vi "Dot Edit.vi"() -> ()   [LabVIEW 2019]
uses:
  Classes/Settings/Dot Settings/Dot Settings.lvclass/Dot Settings.ctl
  Classes/Settings/ObjectSettings/ObjectSettings.lvclass/ObjectSettings.ctl
  Classes/Settings/Dot Settings/Dot Settings.lvclass
  C:/Users/Albro/Documents/GitHub/AFM-Lithography/lvsrc/Classes/Settings/ObjectSettings/ObjectSettings.lvclass
  Classes/Settings/Setting Database/Setting Database.lvclass
  Classes/Settings/Setting Database/Typedefs/PrivateEvents--Setting Database.CopyActiveDotToAll.ctl
  <vilib>/JKI/JKI SMO/SMO/SMO.lvclass
  Classes/Settings/Dot Settings/Accessors/Write Action.vi
  Classes/Settings/ObjectSettings/Accessors/Write Enabled.vi
  Classes/Settings/Dot Settings/Accessors/Read Action.vi
  Classes/Settings/ObjectSettings/Accessors/Read Enabled.vi
panel:
  in  "Save Default":bool
  in  "Copy to All":bool
  in  "Action":u16(ring) caption="Ring" items=["Current Voltage", "Quantum Dot"]
  in  "Enabled?":bool=TRUE
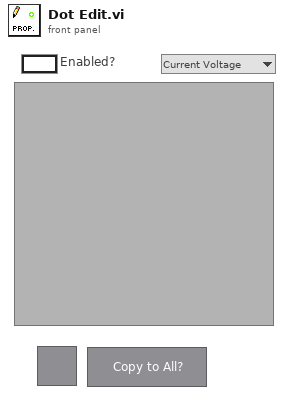
[diagram p1: front panel]
types:
  T1 = enum32{"Invalid", "Standard", "Closed", "Hidden", "Minimized", "Maximized"}
  T2 = enum32{"invalid app kind", "Development System", "Run Time System", "Student Edition", "Embedded LabVIEW", "Evaluation", "Custom"}
  T3 = typedef "Setting Database.lvclass/PrivateEvents--Setting Database.CopyActiveDotToAll.ctl" = bool
  T4 = typedef "Setting Database.lvclass/PublicEvents--Setting Database.NewActiveDot.ctl" = refnum<class "Dot Settings.lvclass">
  T5 = cluster{"Core":cluster{"Current VI Reference":refnum<vi>, "Close Panel on Exit?":bool}, "Active Dot":refnum<class "Dot Settings.lvclass">, "SettingDB":refnum<class "Setting Database.lvclass">, "Subpanels":refnum<vi>[], "Action":u16}
  T6 = cluster{"Current VI Reference":refnum<vi>, "Close Panel on Exit?":bool}
  T7 = typedef "Setting Database.lvclass/PublicEvents--Cluster.ctl" = cluster{"NewActivePath":refnum<user-event>, "PathsUpdated":refnum<user-event>, "RectanglesUpdated":refnum<user-event>, "NewActiveRectangle":refnum<user-event>, "NewActiveFunnel":refnum<user-event>, "FunnelsUpdated":refnum<user-event>, "NewActiveDot":refnum<user-event>, "DotsUpdated":refnum<user-event>}
  T8 = typedef "Dot Settings.lvclass/Action.ctl" = enum16{"IV", "QD"}
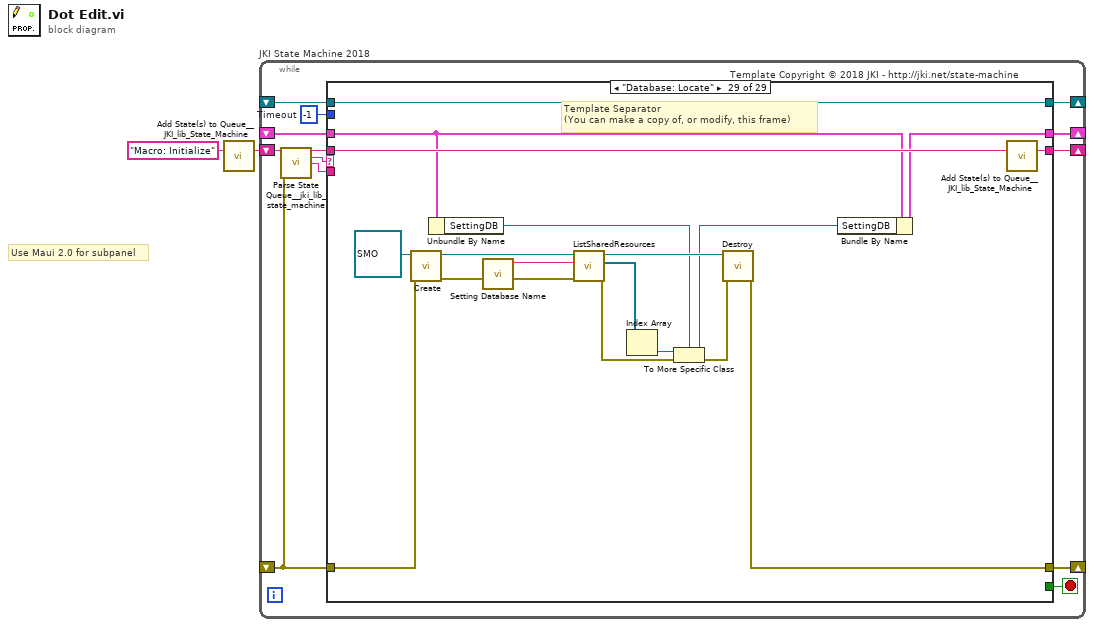
[diagram p0: block diagram]
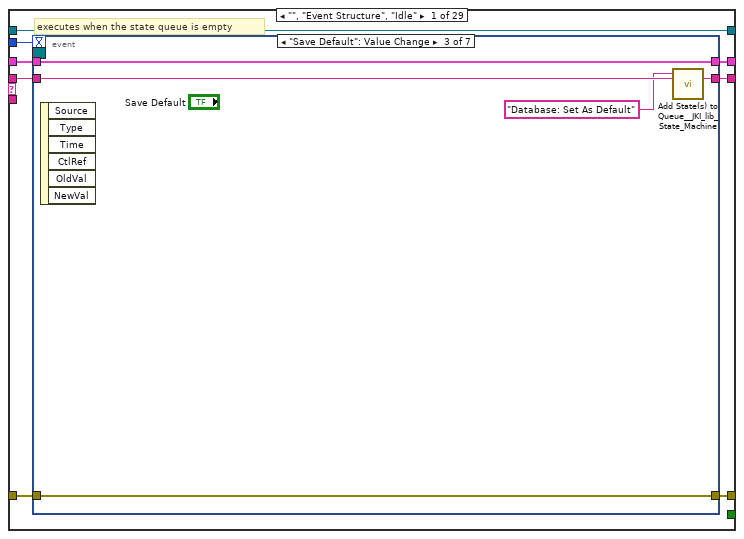
[diagram p2: hidden frame]
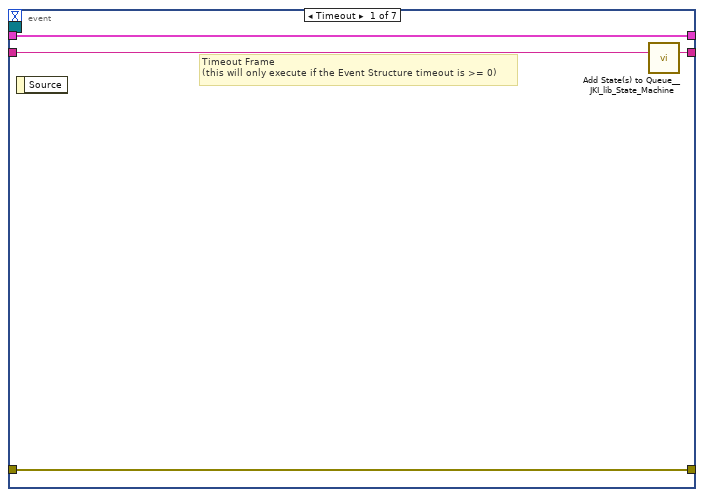
[diagram p3: hidden frame]
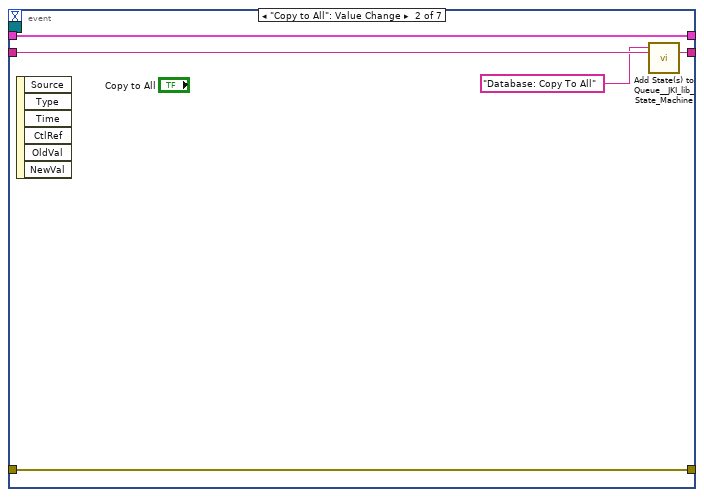
[diagram p4: hidden frame]
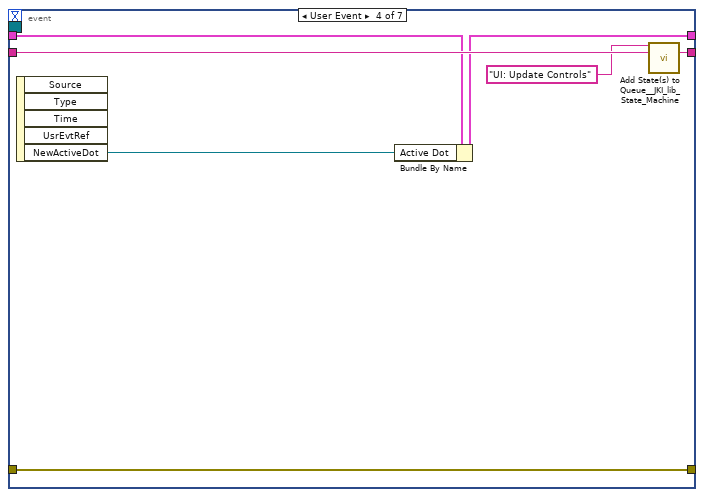
[diagram p5: hidden frame]
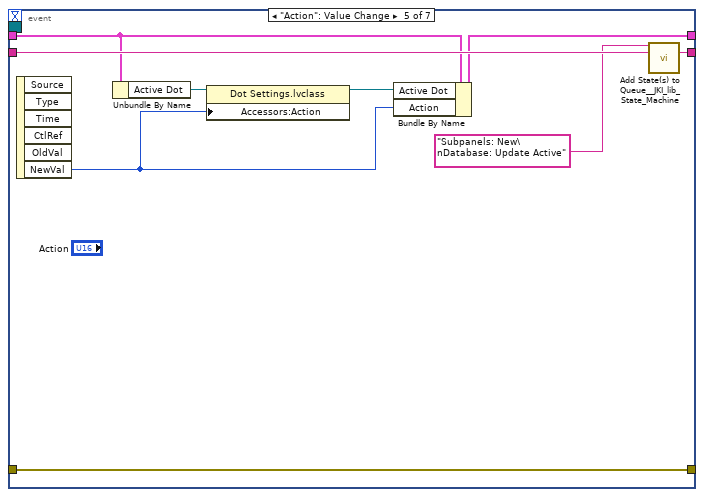
[diagram p6: hidden frame]
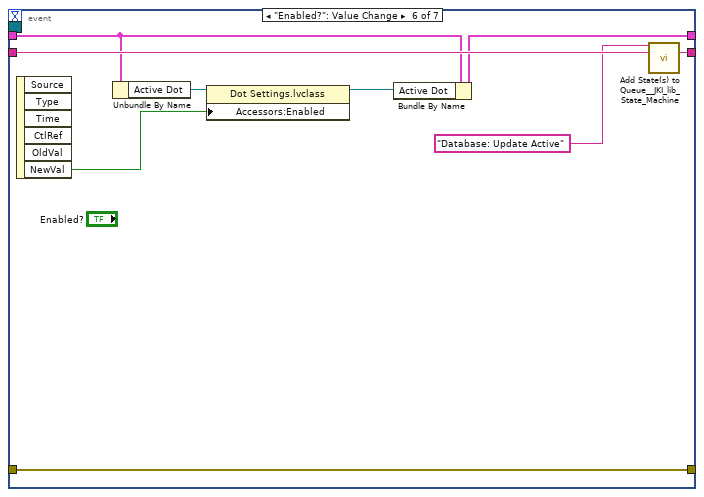
[diagram p7: hidden frame]
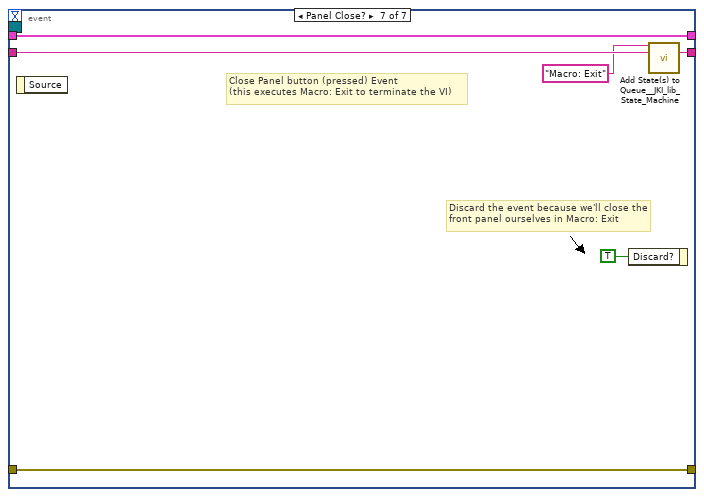
[diagram p8: hidden frame]
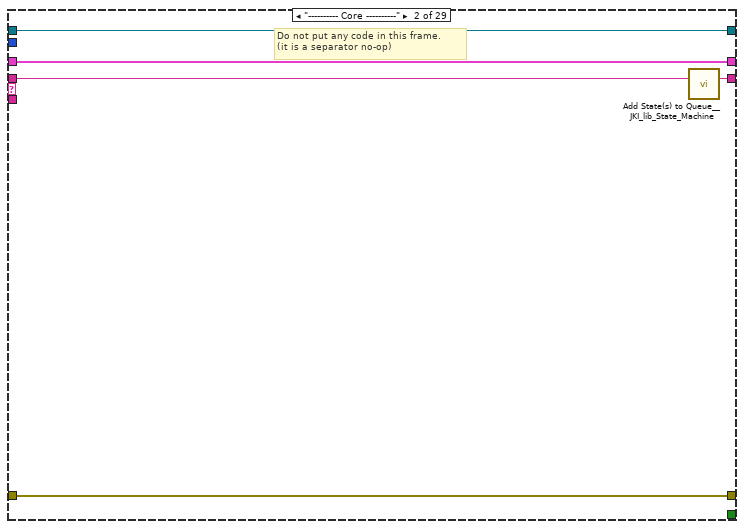
[diagram p9: hidden frame]
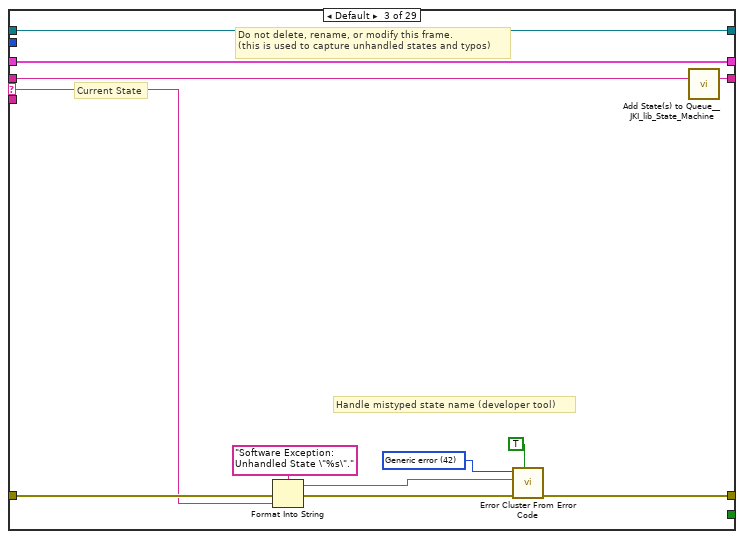
[diagram p10: hidden frame]
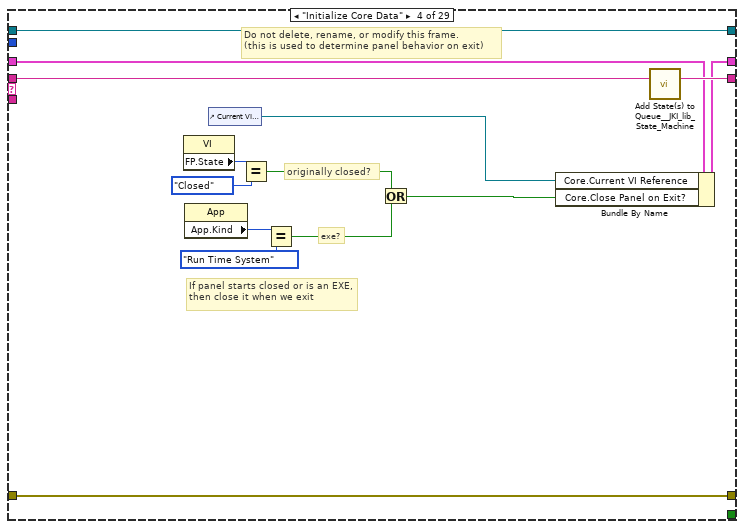
[diagram p11: hidden frame]
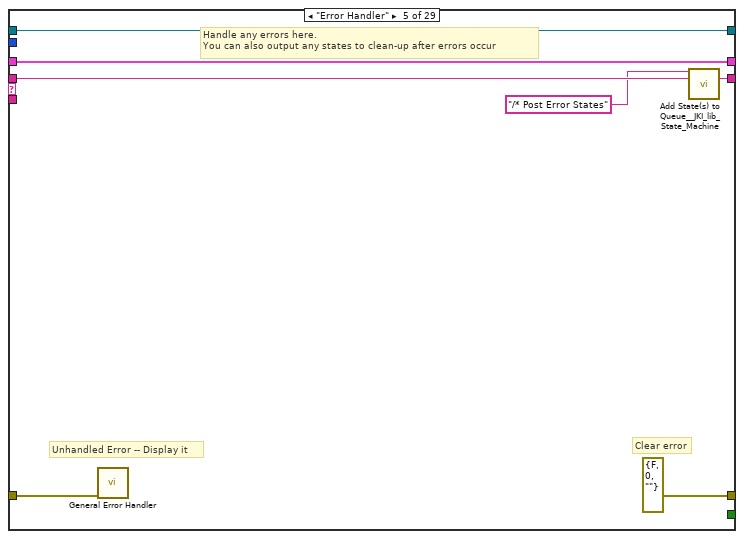
[diagram p12: hidden frame]
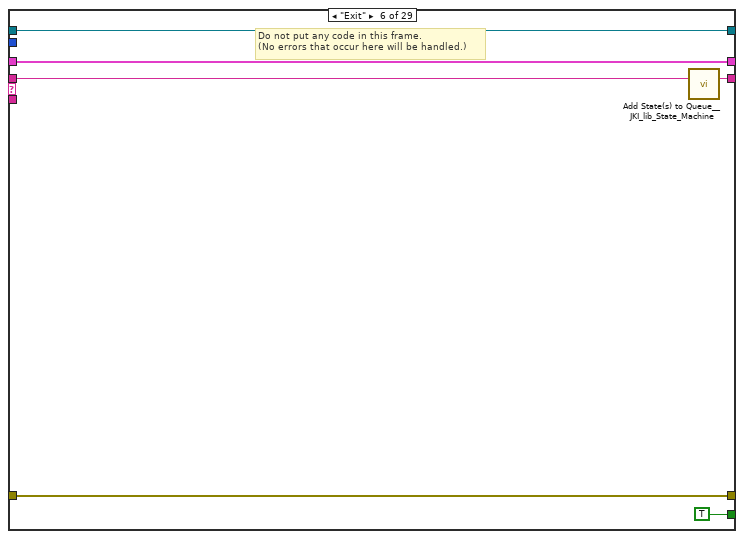
[diagram p13: hidden frame]
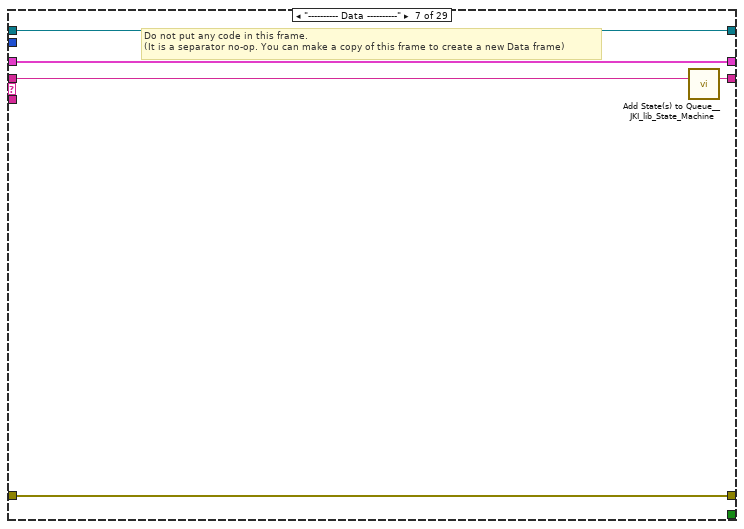
[diagram p14: hidden frame]
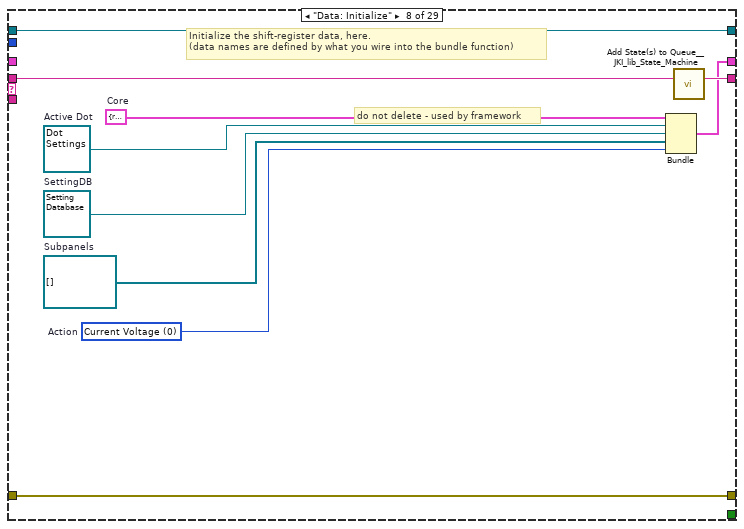
[diagram p15: hidden frame]
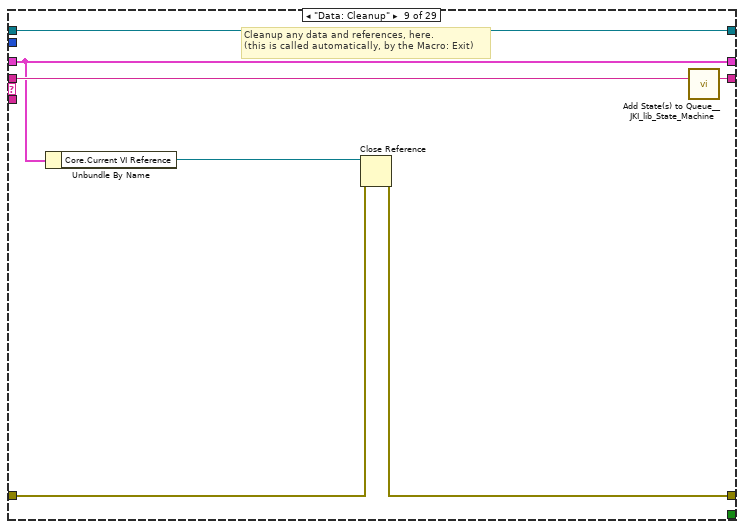
[diagram p16: hidden frame]
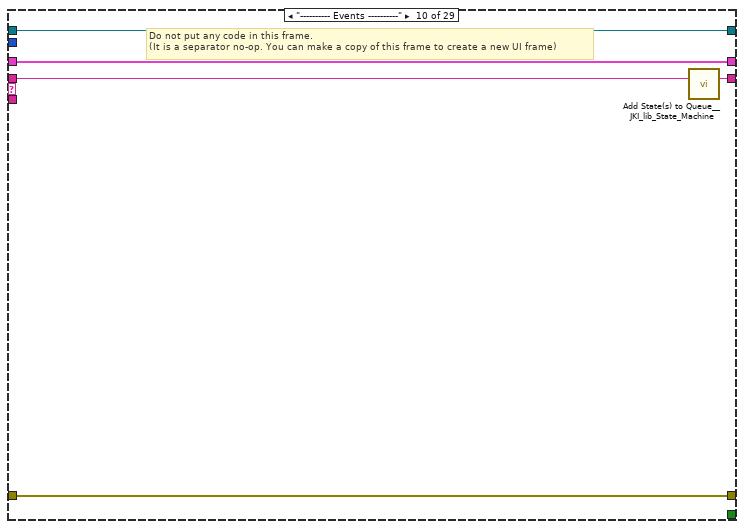
[diagram p17: hidden frame]
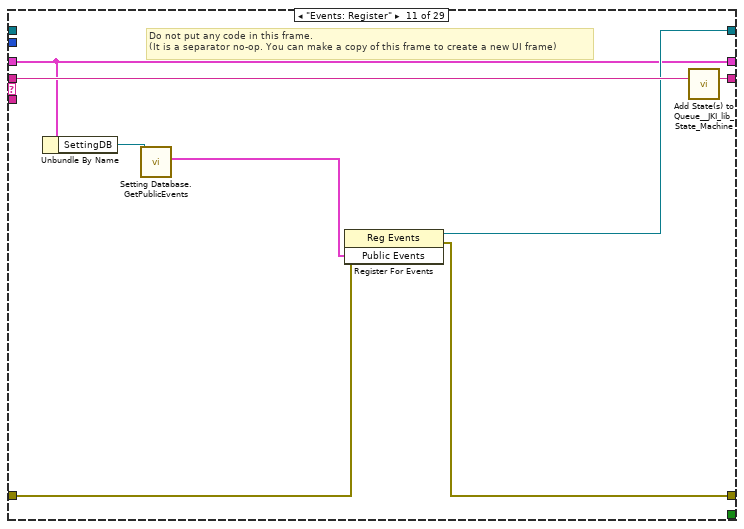
[diagram p18: hidden frame]
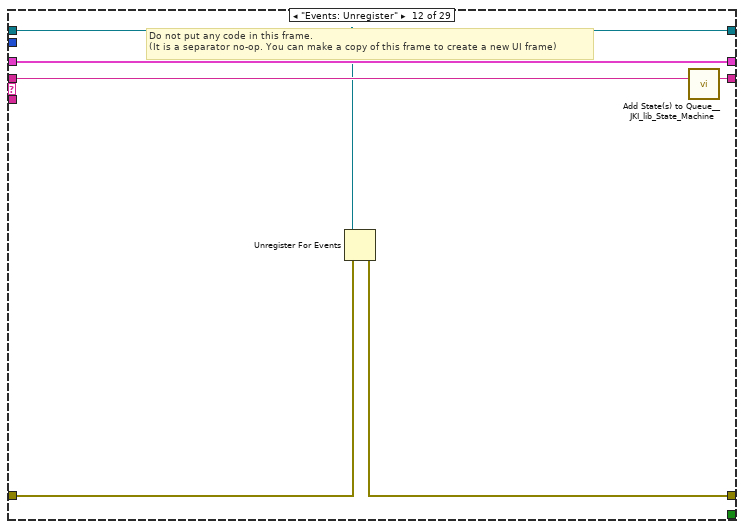
[diagram p19: hidden frame]
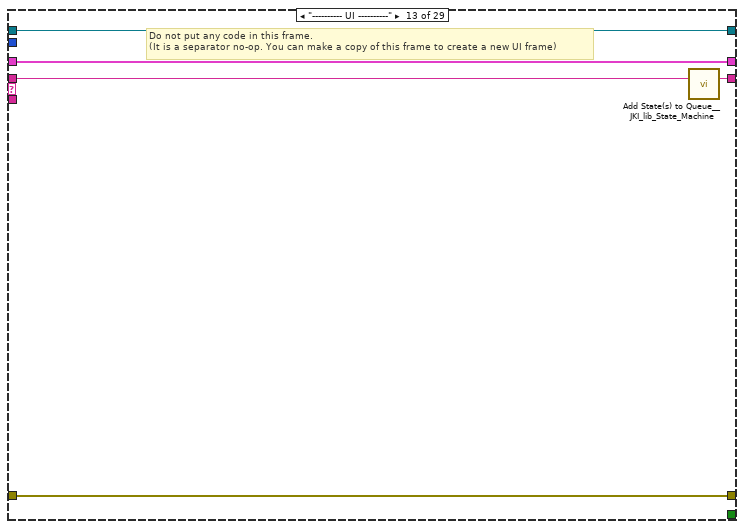
[diagram p20: hidden frame]
diagram:
  # "Use Maui 2.0 for subpanel"
  n1 = call <vilib>:"Add State(s) to Queue__JKI_lib_State_Machine.vi"("State(s) in (\"\")"="Macro: Initialize") -> ("States Out"=w2:string)  [unwired: 14 in]
  n2 = while "JKI State Machine 2018" {
    shift-right: [w8] -> _
    shift-left: _ -> [w7]
    shift-right: [w11] -> _
    shift-left: _ -> [w5]
    shift-right: [w10] -> _
    shift-left: w2 -> [w12]
    shift-right: [w4] -> _
    shift-left: _ -> [w3]
    stop <- w9 stop-if-true
    w6 = -1  # Timeout
    # "Template Copyright © 2018 JKI - http://jki.net/state-machine"
    n3 = call <vilib>:"Parse State Queue__jki_lib_state_machine.vi"("State Queue"=w12, "Error In (no error)"=w5) -> ("Remaining States"=w14:string, "Current State"=w15:string, "Arguments"=w13:string)  [unwired: 11 in]
    n4 = case shown="\"Database: Locate\"" w15 {
      selector: w15 -> [_ _ w75 _ _ _ _ _ _ _ _ _ _ _ _ _ _ _ _ _ _ _ _ _ _ _ _ _ _]
      tunnel: w14 -> [w23 w73 w79 w99 w106 w112 w117 w127 w134 w139 w147 w153 w158 w172 w177 w184 w196 w266 w272 w283 w288 w309 w323 w334 w339 w348 w358 w368 w387]
      tunnel: w13 -> [_ _ _ _ _ _ _ _ _ _ _ _ _ _ _ w179 w190 _ _ _ _ _ _ _ _ _ _ _ _]
      tunnel: w7 -> [w21 w70 w77 w92 w103 w110 w114 _ w129 w136 w143 w151 w155 w166 w175 w182 w192 w263 w269 w280 w285 w302 w320 w332 w336 w344 w354 w365 w371]
      tunnel: [w20 w71 w81 w96 errorcluster {"status"=FALSE, "code"=0, "source"=""} ("error out") w109 w115 w124 w130 w137 w144 w148 w156 w170 w174 w180 w193 w264 w270 w281 w286 w291 w321 w331 w337 w340 w351 w362 w374] -> w11
      tunnel: w5 -> [w19 w71 w80 w96 w102 w109 w115 w124 w131 w137 w140 w149 w156 w170 w174 w181 w194 w264 w270 w281 w286 w297 w321 w330 w337 w341 w350 w361 w373]
      tunnel: [w22 w72 w78 w98 w105 w111 w116 w126 w133 w138 w146 w152 w157 w171 w176 w183 w195 w265 w271 w282 w287 w308 w322 w333 w338 w347 w357 w367 w386] -> w10
      tunnel: [_ _ _ _ _ TRUE _ _ _ _ _ _ _ _ _ _ _ _ _ _ _ _ _ _ _ _ _ _ _] -> w9
      tunnel: [w18 w70 w77 w97 w103 w110 w114 w125 w129 w136 w143 w151 w155 w167 w175 w182 w192 w263 w269 w280 w285 w302 w318 w332 w336 w345 w355 w366 w372] -> w8
      tunnel: w6 -> [w17 _ _ _ _ _ _ _ _ _ _ _ _ _ _ _ _ _ _ _ _ _ _ _ _ _ _ _ _]
      tunnel: [w16 w69 w74 w86 w100 w107 w113 w119 w128 w135 w145 w150 w154 w169 w173 w178 w189 w262 w267 w273 w284 w299 w316 w328 w335 w346 w356 w359 w370] -> w4
      tunnel: w3 -> [w16 w69 w74 w86 w100 w107 w113 w119 w128 w135 _ w150 w154 w169 w173 w178 w189 w262 w267 w273 w284 w299 w316 w328 w335 w346 w356 w359 w370]
      frame "", "Event Structure", "Idle" {
        # "executes when the state queue is empty"
        n5 = event shown="[2] \"Save Default\": Value Change" {
          selector: w16 -> [_ _ _ _ _ _ _]
          dyn-events: _ -> [_ _ _ _ _ _ _]
          timeout: w17 -> [_ _ _ _ _ _ _]
          tunnel: w23 -> [w27 w32 w37 w44 w53 w62 w68]
          tunnel: [w26 w31 w36 w43 w52 w61 w67] -> w22
          tunnel: w21 -> [w24 w29 w34 w41 w47 w55 w65]
          tunnel: [w25 w30 w35 w42 w51 w60 w66] -> w20
          tunnel: w19 -> [w25 w30 w35 w42 w51 w60 w66]
          tunnel: [w24 w29 w34 w40 w48 w56 w65] -> w18
          event Timeout {
            # "Timeout Frame\n(this will only execute if the Event Structure timeout is >= 0)"
            n6 = event-data() -> ()  [unwired: 1 in, 1 out]
            n7 = call <vilib>:"Add State(s) to Queue__JKI_lib_State_Machine.vi"("State(s) in (\"\")"=w27) -> ("States Out"=w26:string)  [unwired: 14 in]
          }
          event "Copy to All": Value Change {
            n8 = event-data() -> ()  [unwired: 1 in, 6 out]
            n9 = call <vilib>:"Add State(s) to Queue__JKI_lib_State_Machine.vi"("State(s) in Front (\"\")"="Database: Copy To All", "State(s) in (\"\")"=w32) -> ("States Out"=w31:string)  [unwired: 13 in]
          }
          event "Save Default": Value Change {
            n10 = event-data() -> ()  [unwired: 1 in, 6 out]
            n11 = call <vilib>:"Add State(s) to Queue__JKI_lib_State_Machine.vi"("State(s) in Front (\"\")"="Database: Set As Default", "State(s) in (\"\")"=w37) -> ("States Out"=w36:string)  [unwired: 13 in]
          }
          event User Event {
            n12 = event-data() -> ("NewActiveDot"=w39:T4)  [unwired: 1 in, 4 out]
            n13 = Bundle By Name(cluster=w41, "Active Dot"=w39) -> (w40:T5)
            n14 = call <vilib>:"Add State(s) to Queue__JKI_lib_State_Machine.vi"("State(s) in Front (\"\")"="UI: Update Controls", "State(s) in (\"\")"=w44) -> ("States Out"=w43:string)  [unwired: 13 in]
          }
          event "Action": Value Change {
            n15 = event-data() -> ("NewVal"=w45:u16)  [unwired: 1 in, 5 out]
            n16 = Unbundle By Name(w47) -> ("Active Dot"=w49:refnum<class "Dot Settings.lvclass">)
            n17 = property class="Dot Settings.lvclass"(reference=w49, "Accessors:Action"=w45) -> (reference out=w46:refnum<class "Dot Settings.lvclass">)  [unwired: 1 in, 1 out]
            n18 = Bundle By Name(cluster=w47, "Active Dot"=w46, "Action"=w45) -> (w48:T5)
            n19 = call <vilib>:"Add State(s) to Queue__JKI_lib_State_Machine.vi"("State(s) in Front (\"\")"="Subpanels: New\nDatabase: Update Active", "State(s) in (\"\")"=w53) -> ("States Out"=w52:string)  [unwired: 13 in]
          }
          event "Enabled?": Value Change {
            n20 = event-data() -> ("NewVal"=w57:bool)  [unwired: 1 in, 5 out]
            n21 = Unbundle By Name(w55) -> ("Active Dot"=w58:refnum<class "Dot Settings.lvclass">)
            n22 = property class="Dot Settings.lvclass"(reference=w58, "Accessors:Enabled"=w57) -> (reference out=w54:refnum<class "Dot Settings.lvclass">)  [unwired: 1 in, 1 out]
            n23 = Bundle By Name(cluster=w55, "Active Dot"=w54) -> (w56:T5)
            n24 = call <vilib>:"Add State(s) to Queue__JKI_lib_State_Machine.vi"("State(s) in Front (\"\")"="Database: Update Active", "State(s) in (\"\")"=w62) -> ("States Out"=w61:string)  [unwired: 13 in]
          }
          event Panel Close? {
            # "Discard the event because we'll close the front panel ourselves in Macro: Exit"
            # "Close Panel button (pressed) Event\n(this executes Macro: Exit to terminate the VI)"
            n25 = event-data() -> ()  [unwired: 1 in, 1 out]
            n26 = event-data("Discard?"=TRUE) -> ()  [unwired: 1 in, 1 out]
            n27 = call <vilib>:"Add State(s) to Queue__JKI_lib_State_Machine.vi"("State(s) in Front (\"\")"="Macro: Exit", "State(s) in (\"\")"=w68) -> ("States Out"=w67:string)  [unwired: 13 in]
          }
        }
      }
      frame "---------- Core ----------" {
        # "Do not put any code in this frame.\n(it is a separator no-op)"
        n28 = call <vilib>:"Add State(s) to Queue__JKI_lib_State_Machine.vi"("State(s) in (\"\")"=w73) -> ("States Out"=w72:string)  [unwired: 14 in]
      }
      frame Default {
        w84 = 42 items=["No error", "Argument error", "Memory is full", "Out of zone", "End of file", "File already open", "Generic file I/O error", "File not found", "File permission error", "Disk is full", "Duplicate path", "Too many files open", "System feature not enabled", "Resource file not found", "Cannot add resource", "Resource not found", "Image not found", "Image memory error", "Pen does not exist", "Config type invalid", "Config token not found", "Config parse error", "Config memory error", "Bad external code format", "Bad external code offset", "External code not present", "Null window", "Destroy window error", "Null menu", "Print aborted", "Bad print record", "Print driver error", "Windows error during printing", "Memory error during printing", "Print dialog error", "Generic print error", "Invalid device refnum", "Device not found", "Device parameter error", "Device unit error", "Cannot open device", "Device call aborted", "Generic error", "Cancelled by user", "Object ID too low", "Object ID too high", "Object not in heap", "Unknown heap", "Unknown object (invalid DefProc)", "Unknown object (DefProc not in table)", "Message out of range", "Invalid (null) method", "Unknown message", "Manager call not supported", "Bad address", "Network operation in progress", "Network operation timed out", "Connection is busy", "Network attribute not supported", "Network error", "Address in use", "System out of memory", "Connection aborted", "Connection refused", "Not connected", "Already connected", "Connection closed", "Initialization error (interapplication manager)", "Bad occurrence", "Wait on unbound occurrence handler", "Occurrence queue overflow", "Datalog type conflict", "Unused", "Unrecognized type (interapplication manager)", "Memory corrupt", "Failed to make temporary DLL", "Old CIN version", "Drag socket not found", "Failed to load drop-object", "Failed to register OLE object", "Failed to release OLE object", "Format specifier type mismatch", "Unknown format specifier", "Too few format specifiers", "Too many format specifiers", "Scan failed", "Newer CIN version", "Error converting to variant", "Runtime menu error", "Password tampered", "Variant attribute not found", "Incompatible variant data type", "Event data is not available", "Event Store is not present", "Occurrence is not found", "Event Queue is not created", "Event info is not available", "Refnum passed is NULL", "Error retrieving Class GUID", "Error retrieving CoClass GUID", "Error retrieving TypeLib GUID.", "Bad built application magic bytes.", "Specific driver is different from the specific driver associated with the Logical Name.", "There is no session opened to the class driver.", "Max Error", "MAX - Error with config objects", "MAX - Error loading configuration", "MAX - Group not supported"]
        # "Current State"
        # "Do not delete, rename, or modify this frame.\n(this is used to capture unhandled states and typos)"
        # "Handle mistyped state name (developer tool)"
        n29 = Format Into String(format string="Software Exception: Unhandled State \"%s\"." ("message"), error in=w80, w75) -> (resulting string=w83:string, error out=w82:errorcluster)  [unwired: 1 in]
        n30 = call <vilib>:"Error Cluster From Error Code.vi"("show call chain? (False)"=TRUE, "error in (no error)"=w82, "error message (\"\")"=w83, "error code (0)"=w84) -> ("error out"=w81:errorcluster)  [unwired: 5 in]
        n31 = call <vilib>:"Add State(s) to Queue__JKI_lib_State_Machine.vi"("State(s) in (\"\")"=w79) -> ("States Out"=w78:string)  [unwired: 14 in]
      }
      frame "Initialize Core Data" {
        # "Do not delete, rename, or modify this frame.\n(this is used to determine panel behavior on exit)"
        # "originally closed?"
        # "exe?"
        # "If panel starts closed or is an EXE, then close it when we exit"
        n32 = property class="VI"() -> ("FP.State"=w89:T1)  [unwired: 2 in, 2 out]
        n33 = property class="App"() -> ("App.Kind"=w95:T2)  [unwired: 2 in, 2 out]
        n34 = control-ref of="Current VI Reference"() -> (w90:refnum<vi>)
        n35 = Equal?(x=w89, y=T1."Closed" ("Front Panel Window:State")) -> (x = y?=w87:bool)
        n36 = Equal?(x=w95, y=T2."Run Time System" ("Application:Kind")) -> (x = y?=w93:bool)
        n37 = Or(x=w87, y=w93) -> (x .or. y?=w91:bool)
        n38 = Bundle By Name(cluster=w92, "Core.Current VI Reference"=w90, "Core.Close Panel on Exit?"=w91) -> (w97:T5)
        n39 = call <vilib>:"Add State(s) to Queue__JKI_lib_State_Machine.vi"("State(s) in (\"\")"=w99) -> ("States Out"=w98:string)  [unwired: 14 in]
      }
      frame "Error Handler" {
        # "Unhandled Error -- Display it"
        # "Handle any errors here.\nYou can also output any states to clean-up after errors occur"
        # "Clear error"
        n40 = call <vilib>:"General Error Handler.vi"("error in (no error)"=w102) -> ()  [unwired: 10 in, 5 out]
        n41 = call <vilib>:"Add State(s) to Queue__JKI_lib_State_Machine.vi"("State(s) in Front (\"\")"="/* Post Error States", "State(s) in (\"\")"=w106) -> ("States Out"=w105:string)  [unwired: 13 in]
      }
      frame "Exit" {
        # "Do not put any code in this frame.\n(No errors that occur here will be handled.)"
        n42 = call <vilib>:"Add State(s) to Queue__JKI_lib_State_Machine.vi"("State(s) in (\"\")"=w112) -> ("States Out"=w111:string)  [unwired: 14 in]
      }
      frame "---------- Data ----------" {
        # "Do not put any code in this frame.\n(It is a separator no-op. You can make a copy of this frame to create a new Data frame)"
        n43 = call <vilib>:"Add State(s) to Queue__JKI_lib_State_Machine.vi"("State(s) in (\"\")"=w117) -> ("States Out"=w116:string)  [unwired: 14 in]
      }
      frame "Data: Initialize" {
        w118 = u16 0 items=["Current Voltage", "Quantum Dot"]  # Action
        w120 = refnum<class "Setting Database.lvclass"> refnum  # SettingDB
        w121 = refnum<class "Dot Settings.lvclass"> refnum  # Active Dot
        w122 = refnum<vi>[] []  # Subpanels
        w123 = T6 {"Current VI Reference"=refnum, "Close Panel on Exit?"=FALSE}  # Core
        # "do not delete - used by framework"
        # "Initialize the shift-register data, here.\n(data names are defined by what you wire into the bundle function)"
        n44 = Bundle("Core"=w123, "Active Dot"=w121, "SettingDB"=w120, "Subpanels"=w122, "Action"=w118) -> (w125:T5)  [unwired: 1 in]
        n45 = call <vilib>:"Add State(s) to Queue__JKI_lib_State_Machine.vi"("State(s) in (\"\")"=w127) -> ("States Out"=w126:string)  [unwired: 14 in]
      }
      frame "Data: Cleanup" {
        # "Cleanup any data and references, here.\n(this is called automatically, by the Macro: Exit)"
        n46 = Unbundle By Name(w129) -> ("Core.Current VI Reference"=w132:refnum<vi>)
        n47 = Close Reference(reference=w132, error in (no error)=w131) -> (error out=w130:errorcluster)
        n48 = call <vilib>:"Add State(s) to Queue__JKI_lib_State_Machine.vi"("State(s) in (\"\")"=w134) -> ("States Out"=w133:string)  [unwired: 14 in]
      }
      frame "---------- Events ----------" {
        # "Do not put any code in this frame.\n(It is a separator no-op. You can make a copy of this frame to create a new UI frame)"
        n49 = call <vilib>:"Add State(s) to Queue__JKI_lib_State_Machine.vi"("State(s) in (\"\")"=w139) -> ("States Out"=w138:string)  [unwired: 14 in]
      }
      frame "Events: Register" {
        # "Do not put any code in this frame.\n(It is a separator no-op. You can make a copy of this frame to create a new UI frame)"
        n50 = Unbundle By Name(w143) -> ("SettingDB"=w142:refnum<class "Setting Database.lvclass">)
        n51 = call "Setting Database.GetPublicEvents.vi"("Setting Database"=w142) -> ("Public Events"=w141:T7)  [unwired: 8 in, 2 out]
        n52 = register-events(error in=w140, w141) -> (reference out=w145:refnum<event-registration>, error out=w144:errorcluster)  [unwired: 1 in]
        n53 = call <vilib>:"Add State(s) to Queue__JKI_lib_State_Machine.vi"("State(s) in (\"\")"=w147) -> ("States Out"=w146:string)  [unwired: 14 in]
      }
      frame "Events: Unregister" {
        # "Do not put any code in this frame.\n(It is a separator no-op. You can make a copy of this frame to create a new UI frame)"
        n54 = Unregister For Events(event registration refnum=w150, error in=w149) -> (error out=w148:errorcluster)
        n55 = call <vilib>:"Add State(s) to Queue__JKI_lib_State_Machine.vi"("State(s) in (\"\")"=w153) -> ("States Out"=w152:string)  [unwired: 14 in]
      }
      frame "---------- UI ----------" {
        # "Do not put any code in this frame.\n(It is a separator no-op. You can make a copy of this frame to create a new UI frame)"
        n56 = call <vilib>:"Add State(s) to Queue__JKI_lib_State_Machine.vi"("State(s) in (\"\")"=w158) -> ("States Out"=w157:string)  [unwired: 14 in]
      }
      frame "UI: Update Controls" {
        # "Do not put any code in this frame.\n(It is a separator no-op. You can make a copy of this frame to create a new UI frame)"
        n57 = Unbundle By Name(w166) -> ("Action"=w164:u16, "Active Dot"=w168:refnum<class "Dot Settings.lvclass">)
        n58 = property class="Dot Settings.lvclass"(reference=w168) -> ("Accessors:Action"=w165:T8, "Accessors:Enabled"=w159:bool)  [unwired: 1 in, 2 out]
        n59 = Equal?(x=w164, y=w165) -> (x = y?=w163:bool)
        n60 = local write "Action"(w165) -> ()
        n61 = local write "Enabled?"(w159) -> ()
        n62 = Bundle By Name(cluster=w166, "Action"=w165) -> (w167:T5)
        n63 = Select(t="", s=w163, f="Subpanels: New" ("State(s) in Front (\"\")")) -> (s? t:f=w161:string)
        n64 = call <vilib>:"Add State(s) to Queue__JKI_lib_State_Machine.vi"("State(s) in Front (\"\")"=w161, "State(s) in (\"\")"=w172) -> ("States Out"=w171:string)  [unwired: 13 in]
      }
      frame "UI: Initialize" {
        # "Initialize the User Interface, here.\n(this is called automatically, by the Macro: Init)"
        n65 = call <vilib>:"Add State(s) to Queue__JKI_lib_State_Machine.vi"("State(s) in (\"\")"=w177) -> ("States Out"=w176:string)  [unwired: 14 in]
      }
      frame "UI: Cursor Set" {
        # "Argument"
        # "Set and Unset Cursor Busy.\n(Usage: \"UI: Cursor Set >> Busy|Idle\")"
        n66 = case shown="\"Idle\", Default" w179 {
          tunnel: w181 -> [w186 w188]
          tunnel: [w185 w187] -> w180
          frame "Idle", Default {
            n67 = call <vilib>:"Unset Busy.vi"("error in (no error)"=w186) -> ("error out"=w185:errorcluster)  [unwired: 10 in]
          }
          frame "Busy" {
            n68 = call <vilib>:"Set Busy.vi"("error in (no error)"=w188) -> ("error out"=w187:errorcluster)  [unwired: 9 in, 1 out]
          }
        }
        n69 = call <vilib>:"Add State(s) to Queue__JKI_lib_State_Machine.vi"("State(s) in (\"\")"=w184) -> ("States Out"=w183:string)  [unwired: 14 in]
      }
      frame "UI: Front Panel State" {
        # "Argument"
        # "Set Front Panel Open or Closed\n(Usage: \"UI: Front Panel State >> Open|Close\")"
        n70 = Unbundle By Name(w192) -> ("Core.Current VI Reference"=w191:refnum<vi>)
        n71 = case shown="\"Minimize\", \"Minimized\"" w190 {
          tunnel: w194 -> [w202 w217 w228 w241 w254]
          tunnel: [w204 w218 w230 w243 w256] -> w193
          tunnel: w191 -> [w203 w215 w229 w242 w255]
          frame "Open", "Standard", Default {
            w197 = T1."Standard" ("State")
            n72 = property class="VI"(reference=w203, error in=w202) -> (reference out=w200:refnum<vi>, error out=w201:errorcluster, "FP.State"=w199:T1)
            n73 = Not Equal?(x=w199, y=w197) -> (x != y?=w198:bool)
            n74 = case shown="True" w198 {
              tunnel: [w208 w210] -> w204
              tunnel: w201 -> [w207 w210]
              tunnel: w200 -> [w206 _]
              tunnel: w197 -> [w205 _]
              frame True {
                n75 = invoke class="VI" method="FP.Open"(reference=w206, error in=w207, "Activate"=TRUE, "State"=w205) -> (error out=w208:errorcluster)  [unwired: 1 in, 4 out]
              }
              frame False {
              }
            }
          }
          frame "Close", "Closed" {
            n76 = property class="VI"(reference=w215, error in=w217) -> (reference out=w214:refnum<vi>, error out=w216:errorcluster, "FP.State"=w212:T1)
            n77 = Not Equal?(x=w212, y=T1."Closed" ("Front Panel Window:State")) -> (x != y?=w211:bool)
            n78 = case shown="True" w211 {
              tunnel: [w219 w222] -> w218
              tunnel: w216 -> [w219 w221]
              tunnel: w214 -> [_ w220]
              frame False {
              }
              frame True {
                n79 = invoke class="VI" method="FP.Close"(reference=w220, error in=w221) -> (error out=w222:errorcluster)  [unwired: 1 in, 2 out]
              }
            }
          }
          frame "Hidden", "Hide" {
            w223 = T1."Hidden" ("State")
            n80 = property class="VI"(reference=w229, error in=w228) -> (reference out=w226:refnum<vi>, error out=w227:errorcluster, "FP.State"=w225:T1)
            n81 = Not Equal?(x=w225, y=w223) -> (x != y?=w224:bool)
            n82 = case shown="True" w224 {
              tunnel: [w234 w235] -> w230
              tunnel: w227 -> [w233 w235]
              tunnel: w226 -> [w232 _]
              tunnel: w223 -> [w231 _]
              frame True {
                n83 = invoke class="VI" method="FP.Open"(reference=w232, error in=w233, "State"=w231) -> (error out=w234:errorcluster)  [unwired: 2 in, 4 out]
              }
              frame False {
              }
            }
          }
          frame "Minimize", "Minimized" {
            w236 = T1."Minimized" ("State")
            n84 = property class="VI"(reference=w242, error in=w241) -> (reference out=w239:refnum<vi>, error out=w240:errorcluster, "FP.State"=w238:T1)
            n85 = Not Equal?(x=w238, y=w236) -> (x != y?=w237:bool)
            n86 = case shown="True" w237 {
              tunnel: [w247 w248] -> w243
              tunnel: w240 -> [w246 w248]
              tunnel: w239 -> [w245 _]
              tunnel: w236 -> [w244 _]
              frame True {
                n87 = invoke class="VI" method="FP.Open"(reference=w245, error in=w246, "State"=w244) -> (error out=w247:errorcluster)  [unwired: 2 in, 4 out]
              }
              frame False {
              }
            }
          }
          frame "Maximize", "Maximized" {
            w249 = T1."Maximized" ("State")
            n88 = property class="VI"(reference=w255, error in=w254) -> (reference out=w252:refnum<vi>, error out=w253:errorcluster, "FP.State"=w251:T1)
            n89 = Not Equal?(x=w251, y=w249) -> (x != y?=w250:bool)
            n90 = case shown="True" w250 {
              tunnel: [w260 w261] -> w256
              tunnel: w253 -> [w259 w261]
              tunnel: w252 -> [w258 _]
              tunnel: w249 -> [w257 _]
              frame True {
                n91 = invoke class="VI" method="FP.Open"(reference=w258, error in=w259, "State"=w257) -> (error out=w260:errorcluster)  [unwired: 2 in, 4 out]
              }
              frame False {
              }
            }
          }
        }
        n92 = call <vilib>:"Add State(s) to Queue__JKI_lib_State_Machine.vi"("State(s) in (\"\")"=w196) -> ("States Out"=w195:string)  [unwired: 14 in]
      }
      frame "---------- Macro ----------" {
        # "Do not put any code in this frame.\n(It is a separator no-op. You can make a copy of this frame to create a new Macro frame)"
        n93 = call <vilib>:"Add State(s) to Queue__JKI_lib_State_Machine.vi"("State(s) in (\"\")"=w266) -> ("States Out"=w265:string)  [unwired: 14 in]
      }
      frame "Macro: Initialize" {
        # "Initialization Macro\n(This is called once, when the VI starts)"
        n94 = call <vilib>:"Add State(s) to Queue__JKI_lib_State_Machine.vi"("State(s) in Front (\"\")"="Data: Initialize\nInitialize Core Data\nDatabase: Locate\nEvents: Register\nUI: Initialize\nUI: Front Panel State >> Close\nSubpanels: Run VIs\nSubpanels: New", "State(s) in (\"\")"=w272) -> ("States Out"=w271:string)  [unwired: 13 in]
      }
      frame "Macro: Exit" {
        # "Exit Macro\n(This is called once, when the VI exits)"
        n95 = Unbundle By Name(w280) -> ("Core.Close Panel on Exit?"=w279:bool)
        n96 = Select(t="UI: Front Panel State >> Close", s=w279, f="") -> (s? t:f=w276:string)
        n97 = call <vilib>:"Add State(s) to Queue__JKI_lib_State_Machine.vi"("State(s) in (\"\")"=w276, "State(s) at Back (\"\")"="Subpanels: Stop VIs\nData: Cleanup\nEvents: Unregister\nExit") -> ("States Out"=w274:string)  [unwired: 13 in]
        n98 = call <vilib>:"Add State(s) to Queue__JKI_lib_State_Machine.vi"("State(s) in Front (\"\")"=w274, "State(s) in (\"\")"=w283) -> ("States Out"=w282:string)  [unwired: 13 in]
      }
      frame "---------- Subpanels ----------" {
        # "Template Separator\n(You can make a copy of, or modify, this frame)"
        n99 = call <vilib>:"Add State(s) to Queue__JKI_lib_State_Machine.vi"("State(s) in (\"\")"=w288) -> ("States Out"=w287:string)  [unwired: 14 in]
      }
      frame "Subpanels: New" {
        # "Template Separator\n(You can make a copy of, or modify, this frame)"
        n100 = Unbundle By Name(w302) -> ("Core.Current VI Reference"=w290:refnum<vi>, "Subpanels"=w301:refnum<vi>[], "Action"=w296:u16)
        n101 = control-ref of="Sub Panel"() -> (w307:refnum<vi>)
        n102 = property class="SubPnl"(reference=w307, error in=w297) -> (reference out=w304:refnum<vi>, error out=w295:errorcluster, "InsertedVI"=w306:refnum<vi>)
        n103 = Index Array(array=w301, index=w296) -> (element=w300:refnum<vi>)
        n104 = Not A Number/Path/Refnum?(number/path/refnum=w306) -> (NaN/Path/Refnum?=w305:bool)
        n105 = call <userlib>:"MGI Defer Panel Updates.vi"("Error In"=w295, "Defer Updates?"=TRUE, "VI Reference (Caller)"=w290) -> ("Error Out"=w294:errorcluster)  [unwired: 8 in]
        n106 = case shown="False" w305 {
          tunnel: w304 -> [w313 w315]
          tunnel: [w312 w315] -> w303
          tunnel: w294 -> [w311 w314]
          tunnel: [w310 w314] -> w298
          frame False {
            n107 = invoke class="SubPnl" method="Remove VI"(reference=w313, error in=w311) -> (reference out=w312:refnum<vi>, error out=w310:errorcluster)  [unwired: 1 in, 1 out]
          }
          frame True {
          }
        }
        n108 = invoke class="SubPnl" method="Insert VI"(reference=w303, error in=w298, "VI Ref"=w300) -> (error out=w292:errorcluster)  [unwired: 1 in, 3 out]
        n109 = call <userlib>:"MGI Defer Panel Updates.vi"("Error In"=w292, "Defer Updates?"=FALSE, "VI Reference (Caller)"=w290) -> ("Error Out"=w291:errorcluster)  [unwired: 8 in]
        n110 = call <vilib>:"Add State(s) to Queue__JKI_lib_State_Machine.vi"("State(s) in (\"\")"=w309) -> ("States Out"=w308:string)  [unwired: 14 in]
      }
      frame "Subpanels: Run VIs" {
        # "Your code here.\n(You can make a copy of, or modify, this frame)"
        n111 = for {
          tunnel: path[] [path "../subpanel/subsubpanel/IVCurve Edit.vi", path "../subpanel/subsubpanel/QuantumDot Edit.vi"] -> [w327] mode=indexing
          tunnel: [w324] -> w319 mode=indexing
          n112 = Open VI Reference(vi path=w327) -> (vi reference=w326:refnum<vi>)  [unwired: 5 in, 1 out]
          n113 = invoke class="VI" method="Run VI"(reference=w326, "Wait until done"=FALSE ("Wait Until Done")) -> (reference out=w324:refnum<vi>)  [unwired: 3 in, 4 out]
        }
        n114 = Bundle By Name(cluster=w320, "Subpanels"=w319) -> (w318:T5)
        n115 = call <vilib>:"Add State(s) to Queue__JKI_lib_State_Machine.vi"("State(s) in (\"\")"=w323) -> ("States Out"=w322:string)  [unwired: 14 in]
      }
      frame "Subpanels: Stop VIs" {
        # "Your code here.\n(You can make a copy of, or modify, this frame)"
        n116 = Unbundle By Name(w332) -> ("Subpanels"=w329:refnum<vi>[])
        n117 = Close Reference(reference=w329, error in (no error)=w330) -> (error out=w331:errorcluster)
        n118 = call <vilib>:"Add State(s) to Queue__JKI_lib_State_Machine.vi"("State(s) in (\"\")"=w334) -> ("States Out"=w333:string)  [unwired: 14 in]
      }
      frame "---------- Database ----------" {
        # "Template Separator\n(You can make a copy of, or modify, this frame)"
        n119 = call <vilib>:"Add State(s) to Queue__JKI_lib_State_Machine.vi"("State(s) in (\"\")"=w339) -> ("States Out"=w338:string)  [unwired: 14 in]
      }
      frame "Database: Set As Default" {
        # "Template Separator\n(You can make a copy of, or modify, this frame)"
        n120 = Unbundle By Name(w344) -> ("SettingDB"=w343:refnum<class "Setting Database.lvclass">)
        n121 = call "Setting Database.SetDefaultDot.vi"("error in (no error)"=w341, "Setting Database"=w343) -> ("error out"=w340:errorcluster, "Setting Database out"=w342:refnum<class "Setting Database.lvclass">)  [unwired: 8 in]
        n122 = Bundle By Name(cluster=w344, "SettingDB"=w342) -> (w345:T5)
        n123 = call <vilib>:"Add State(s) to Queue__JKI_lib_State_Machine.vi"("State(s) in (\"\")"=w348) -> ("States Out"=w347:string)  [unwired: 14 in]
      }
      frame "Database: Copy To All" {
        # "Template Separator\n(You can make a copy of, or modify, this frame)"
        n124 = Unbundle By Name(w354) -> ("SettingDB"=w353:refnum<class "Setting Database.lvclass">)
        n125 = call "Setting Database.CopyActiveDotToAll.vi"("error in (no error)"=w350, "CopyActiveDotToAll"=T3 TRUE, "Setting Database"=w353) -> ("error out"=w351:errorcluster, "Setting Database out"=w352:refnum<class "Setting Database.lvclass">)  [unwired: 7 in]
        n126 = Bundle By Name(cluster=w354, "SettingDB"=w352) -> (w355:T5)
        n127 = call <vilib>:"Add State(s) to Queue__JKI_lib_State_Machine.vi"("State(s) in (\"\")"=w358) -> ("States Out"=w357:string)  [unwired: 14 in]
      }
      frame "Database: Update Active" {
        # "Template Separator\n(You can make a copy of, or modify, this frame)"
        n128 = Unbundle By Name(w365) -> ("SettingDB"=w364:refnum<class "Setting Database.lvclass">, "Active Dot"=w360:refnum<class "Dot Settings.lvclass">)
        n129 = call "Setting Database.UpdateActiveDot.vi"("error in (no error)"=w361, "UpdateActiveDot"=w360, "Setting Database"=w364) -> ("error out"=w362:errorcluster, "Setting Database"=w363:refnum<class "Setting Database.lvclass">)  [unwired: 7 in]
        n130 = Bundle By Name(cluster=w365, "SettingDB"=w363) -> (w366:T5)
        n131 = call <vilib>:"Add State(s) to Queue__JKI_lib_State_Machine.vi"("State(s) in (\"\")"=w368) -> ("States Out"=w367:string)  [unwired: 14 in]
      }
      frame "Database: Locate" {
        # "Template Separator\n(You can make a copy of, or modify, this frame)"
        n132 = call <vilib>:"Create.vi"("error in (no error)"=w373, "SMO"=refnum<class "SMO.lvclass"> refnum) -> ("error out"=w382:errorcluster, "SMO out"=w385:refnum<class "SMO.lvclass">)  [unwired: 7 in, 1 out]
        n133 = Unbundle By Name(w371) -> ("SettingDB"=w378:refnum<class "Setting Database.lvclass">)
        n134 = call "Setting Database Name.vi"("error in (no error)"=w382) -> ("error out"=w381:errorcluster, "Name"=w383:string)  [unwired: 9 in]
        n135 = call <vilib>:"ListSharedResources.vi"("error in (no error)"=w381, "Filter (regex|name)"=w383, "SMO in"=w385) -> ("error out"=w376:errorcluster, "Shared Resources"=w380:refnum<class "SMO.lvclass">[], "SMO out"=w384:refnum<class "SMO.lvclass">)  [unwired: 5 in, 1 out]
        n136 = Index Array(array=w380) -> (element=w379:refnum<class "SMO.lvclass">)  [unwired: 1 in]
        n137 = To More Specific Class(target class=w378, reference=w379, error in=w376) -> (specific class reference=w377:refnum<class "Setting Database.lvclass">, error out=w375:errorcluster)
        n138 = call <vilib>:"Destroy.vi"("error in (no error)"=w375, "SMO"=w384) -> ("error out"=w374:errorcluster)  [unwired: 9 in]
        n139 = Bundle By Name(cluster=w371, "SettingDB"=w377) -> (w372:T5)
        n140 = call <vilib>:"Add State(s) to Queue__JKI_lib_State_Machine.vi"("State(s) in (\"\")"=w387) -> ("States Out"=w386:string)  [unwired: 14 in]
      }
    }
  }
